vi "GetFileTree.vi"(6 "patterns":string[](array[string]), 9 "Tree":refnum<vi>, 10 "Open?":bool, 11 "Base Path":path) -> ()   [LabVIEW 2020]
panel:
  out "All Files in Dir":path[](array[path])
  in  "Tree":string(tree)
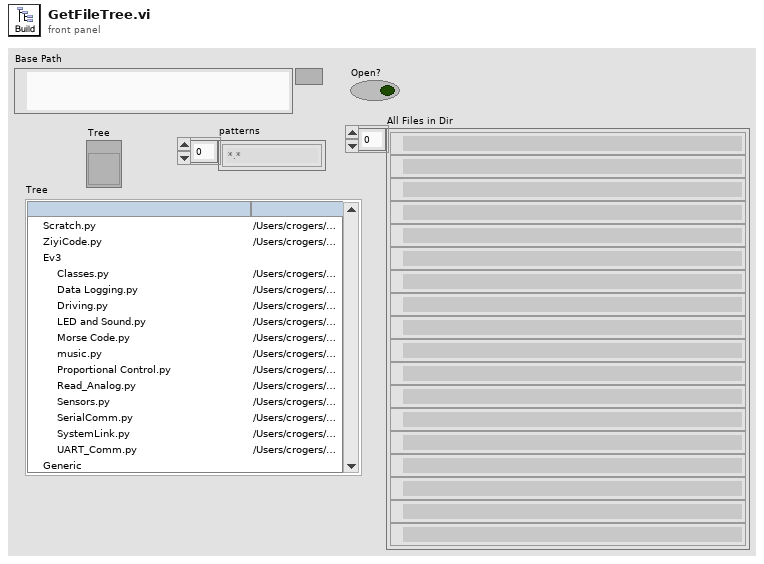
[diagram p1: front panel]
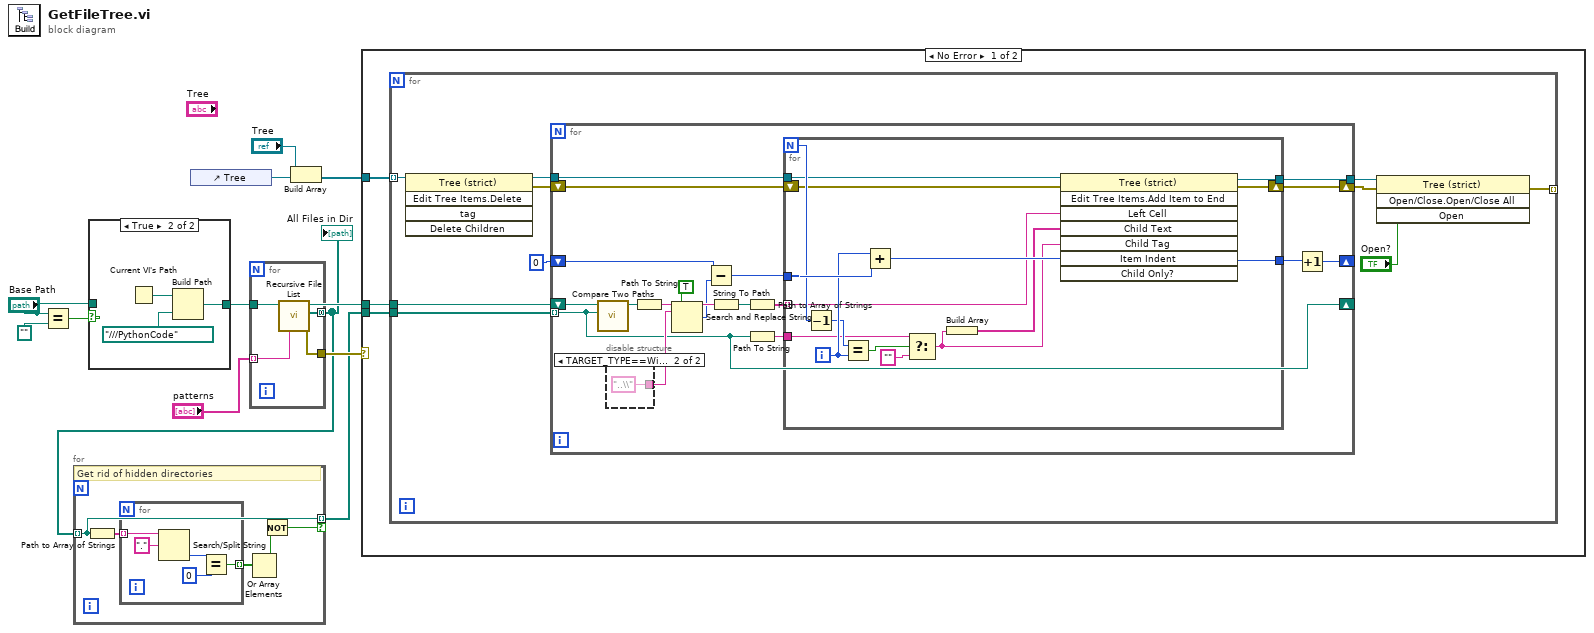
[diagram p0: block diagram]
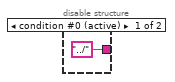
[diagram p3: hidden frame]
diagram:
  n1 = Equal?(x="Base Path", y=path "") -> (x = y?=w9:bool)
  n2 = case shown="True" w9 {
    tunnel: [w12 w13] -> w3
    tunnel: "Base Path" -> [w12 _]
    frame False {
    }
    frame True {
      n3 = Current VI's Path() -> (path=w15:path)
      n4 = Build Path(base path=w15, name or relative path=path "../../../PythonCode") -> (appended path=w13:path)
    }
  }
  n5 = control-ref of="Tree"() -> (w6:refnum<vi>)
  n6 = for {
    tunnel: [w19] -> w2 mode=concatenating
    tunnel: [w18] -> w11
    tunnel: "patterns" -> [w17] mode=indexing
    tunnel: w3 -> [w16]
    n7 = call <vilib>:"Recursive File List.vi"("pattern"=w17, "Folder Path"=w16) -> ("error out"=w18:errorcluster, "All Files in Dir"=w19:path[])  [unwired: 5 in, 3 out]
  }
  "All Files in Dir" <- w2
  n8 = for {
    tunnel: w2 -> [w22] mode=indexing
    tunnel: [w22] -> w1 mode=indexing if=w20
    # "Get rid of hidden directories"
    n9 = Path to Array of Strings(0:w22) -> (2:w24:string[])  [unwired: 1 out]
    n10 = for {
      tunnel: w24 -> [w29] mode=indexing
      tunnel: [w25] -> w23 mode=indexing
      n11 = Search/Split String(string=w29, search string/char (-)=".") -> (offset of match=w27:i32)  [unwired: 1 in, 2 out]
      n12 = Equal?(x=w27, y=0) -> (x = y?=w25:bool)
    }
    n13 = Or Array Elements(Boolean array=w23) -> (logical OR=w21:bool)
    n14 = Not(x=w21) -> (.not. x?=w20:bool)
  }
  n15 = Build Array("Tree", w6) -> (w5:refnum<vi>[])
  n16 = case shown="No Error" w11 {
    tunnel: w5 -> [w32 _]
    tunnel: w1 -> [w31 _]
    tunnel: w3 -> [w30 _]
    frame No Error {
      n17 = for {
        tunnel: w32 -> [w42] mode=indexing
        tunnel: w31 -> [w40]
        tunnel: w30 -> [w39]
        tunnel: [w33] -> _ mode=indexing
        n18 = invoke on="Invoke Node" class="Tree (strict)" method="Edit Tree Items.Delete"(reference=w42) -> (reference out=w38:refnum<vi>, error out=w35:errorcluster)  [unwired: 4 in, 3 out]
        n19 = for {
          tunnel: w40 -> [w48] mode=indexing
          shift-right: [w48] -> _
          shift-left: w39 -> [w61]
          shift-right: [w49] -> _
          shift-left: 0 -> [w51]
          tunnel: w38 -> [w46]
          tunnel: [w45] -> w36
          shift-right: [w43] -> w34
          shift-left: w35 -> [w44]
          n20 = call <vilib>:"Compare Two Paths.vi"("Path 2"=w48, "Path 1"=w61) -> ("Relative Path from 1 to 2"=w53:path)  [unwired: 6 in, 3 out]
          n21 = disable-structure shown="TARGET_TYPE==Windows, Default" {
            disable-tunnel: ["../" ("search string") "..\\" ("search string")] -> w59
            frame condition #0 (active) {
            }
            frame condition #1 {
            }
          }
          n22 = Path To String(path=w53) -> (string=w60:string)
          n23 = Search and Replace String(replace all?=TRUE ("replace all? (F)"), input string=w60, search string=w59) -> (result string=w57:string, number of replacements=w54:i32)  [unwired: 5 in, 2 out]
          n24 = Subtract(x=w51, y=w54) -> (x-y=w52:i32)
          n25 = String To Path(string=w57) -> (path=w56:path)
          n26 = Path to Array of Strings(0:w56) -> (2:w55:string[])  [unwired: 1 out]
          n27 = Path To String(path=w48) -> (string=w47:string)
          n28 = for {
            N -> [w74]
            tunnel: w55 -> [w65] mode=indexing
            tunnel: w52 -> [w77]
            tunnel: [w76] -> w50
            tunnel: w47 -> [w68]
            tunnel: w46 -> [w64]
            tunnel: [w64] -> w45
            shift-right: [w67] -> w43
            shift-left: w44 -> [w66]
            i -> [w75]
            n29 = Decrement(x=w74) -> (x-1=w73:i32)
            n30 = Equal?(x=w73, y=w75) -> (x = y?=w72:bool)
            n31 = Add(x=w75, y=w77) -> (x+y=w76:i32)
            n32 = Select(t=w68, s=w72, f="") -> (s? t:f=w70:string)
            n33 = Build Array(w70) -> (w69:string[])
            n34 = invoke on="Invoke Node" class="Tree (strict)" method="Edit Tree Items.Add Item to End"(reference=w64, error in=w66, "Left Cell"=w65, "Child Text"=w69, "Child Tag"=w70, "Item Indent"=w76) -> (error out=w67:errorcluster)  [unwired: 2 in, 7 out]
          }
          n35 = Increment(x=w50) -> (x+1=w49:i32)
        }
        n36 = invoke on="Invoke Node" class="Tree (strict)" method="Open/Close.Open/Close All"(reference=w36, error in=w34, "Open"="Open?") -> (error out=w33:errorcluster)  [unwired: 1 in, 3 out]
      }
    }
    frame Error {
    }
  }
